vi "Configure Calibration Kit.vi"(7 "Connector type":T1(ring), 8 "error in (no error)":errorcluster, 10 "Cal kit":string, 11 "VNA-ZNB in":refnum<class "VNA-ZNB.lvclass">) -> (0 "error out":errorcluster, 3 "VNA-ZNB out":refnum<class "VNA-ZNB.lvclass">)   [LabVIEW 2020, in "VNA-ZNB.lvclass"]
doc: "Configure the calibration kit to use."
uses:
  VNA-ZNB.lvclass
  C:/Sandbox/Git_Sandbox/WiSpry Test Framework source code (LV20)/WiSpry Test Framework/Instruments/Instrument.lvclass
  Instrument.lvclass/Instrument.ctl
  Instrument.lvclass
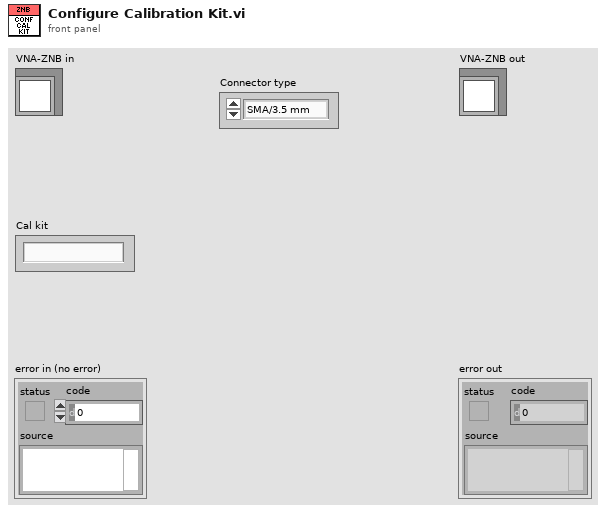
[diagram p1: front panel]
types:
  T1 = enum16{"SMA/3.5 mm", "2.92 mm", "2.4 mm", "1.85 mm", "N 50 Ohm", "N 75 Ohm", "7-16"}
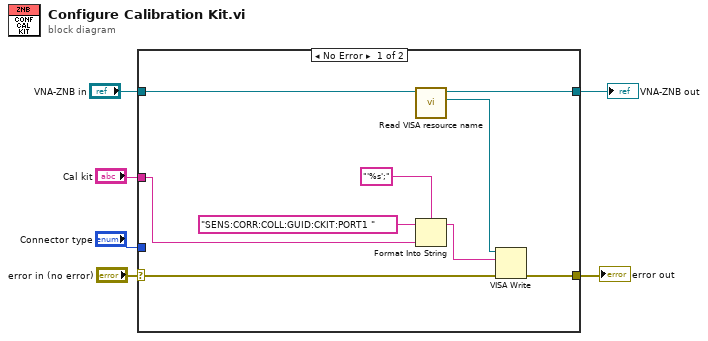
[diagram p0: block diagram]
diagram:
  n1 = case shown="No Error" "error in (no error)" {
    selector: "error in (no error)" -> [w14 w17]
    tunnel: "Cal kit" -> [w15 _]
    tunnel: [w13 w17] -> w4
    tunnel: "VNA-ZNB in" -> [w12 w16]
    tunnel: "Connector type" -> [_ _]
    tunnel: [w11 w16] -> w1
    frame No Error {
      n2 = call "Read VISA resource name.vi"("Instrument in"=w12) -> ("VISA resource name"=w10:refnum<visa-resource-name>, "Instrument out"=w11:refnum<class "VNA-ZNB.lvclass">)  [unwired: 9 in]
      n3 = Format Into String(format string="'%s';", initial string="SENS:CORR:COLL:GUID:CKIT:PORT1 ", w15) -> (resulting string=w7:string)  [unwired: 1 in, 1 out]
      n4 = VISA Write(VISA resource name=w10, write buffer=w7, error in (no error)=w14) -> (error out=w13:errorcluster)  [unwired: 2 out]
    }
    frame Error {
    }
  }
  "error out" <- w4
  "VNA-ZNB out" <- w1
